vi "Zero Pad Removal and Deinterleave.vi"(11 "Input":cdb[](array[numeric])) -> (1 "max index(es)":i32, 2 "Ref":cdb[](array[numeric]), 3 "Data":cdb[](array[numeric]))   [LabVIEW 2014]
doc: "1. Removes zero padding\n2. Deinterleaves data and extracts refrence symbols"
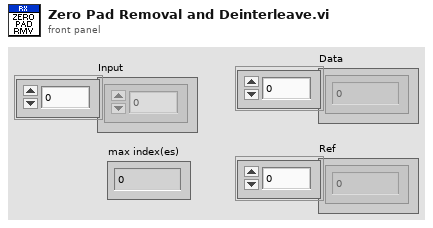
[diagram p1: front panel]
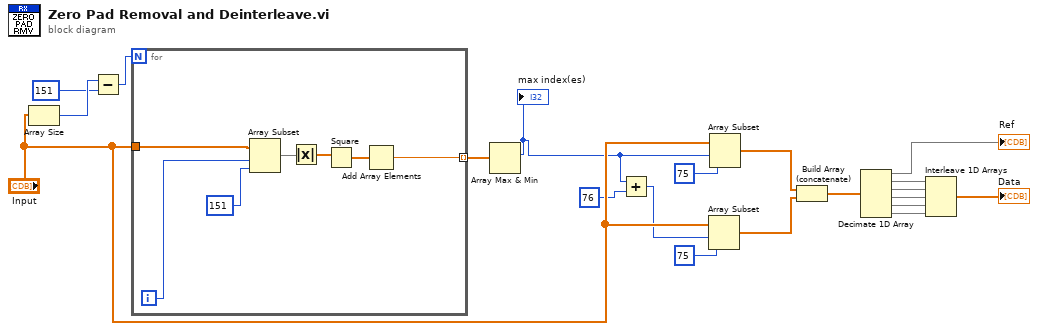
[diagram p0: block diagram]
diagram:
  n1 = Array Size(array="Input") -> (size(s)=w8:i32)
  n2 = Subtract(x=w8, y=151) -> (x-y=w6:i32)
  n3 = for {
    N: w6 -> [_]
    tunnel: "Input" -> [w25]
    tunnel: [w21] -> w5 mode=indexing
    i -> [w27]
    n4 = Array Subset(array=w25, index=w27, length=151) -> (w24:cdb[])
    n5 = Absolute Value(x=w24) -> (abs(x)=w23:dbl[])
    n6 = Square(x=w23) -> (x^2=w22:dbl[])
    n7 = Add Array Elements(numeric array=w22) -> (sum=w21:dbl)
  }
  n8 = Array Max & Min(array=w5) -> (max index (indices)=w3:i32)  [unwired: 3 out]
  "max index(es)" <- w3
  n9 = Add(x=w3, y=76) -> (x+y=w1:i32)
  n10 = Array Subset(array="Input", index=w1, length=75) -> (w13:cdb[])
  n11 = Array Subset(array="Input", index=w3, length=75) -> (w12:cdb[])
  n12 = Build Array (concatenate)(w12, w13) -> (w14:cdb[])
  n13 = Decimate 1D Array(w14) -> (→"Ref":cdb[], w15:cdb[], w16:cdb[], w17:cdb[], w18:cdb[], w19:cdb[])
  n14 = Interleave 1D Arrays(w15, w16, w17, w18, w19) -> (→"Data":cdb[])
